vi "ShowInstrParams.vi"(4 "queue out":refnum<queue>, 6 "user event out":refnum<user-event>, 8 "error in (no error)":errorcluster caption="entrée d'erreur (pas d'erreur)", 10 "InstrParam":string, 11 "Experiment en entrée":refnum<class "Experiment.lvclass"> caption="DNL_LabVIEW Object in") -> (0 "error out":errorcluster caption="sortie d'erreur", 3 "Experiment en sortie":refnum<class "Experiment.lvclass"> caption="DNL_LabVIEW Object out")   [LabVIEW 2019, in "Experiment.lvclass"]
uses:
  Experiment.lvclass
  Experiment.lvclass/Experiment.ctl
  DevicesClass/BaseDevice/BaseDevice.lvclass
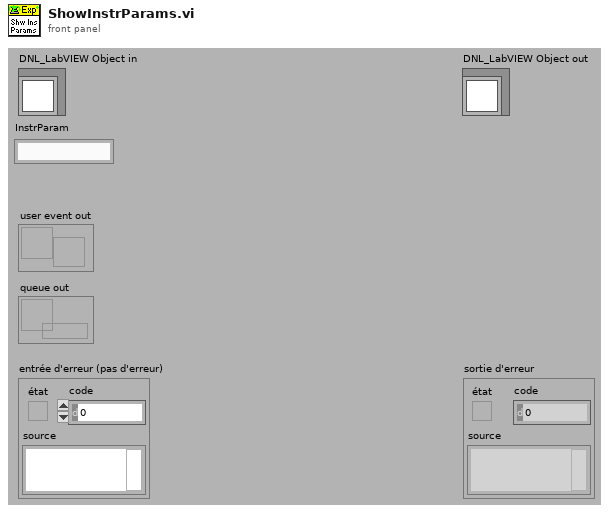
[diagram p1: front panel]
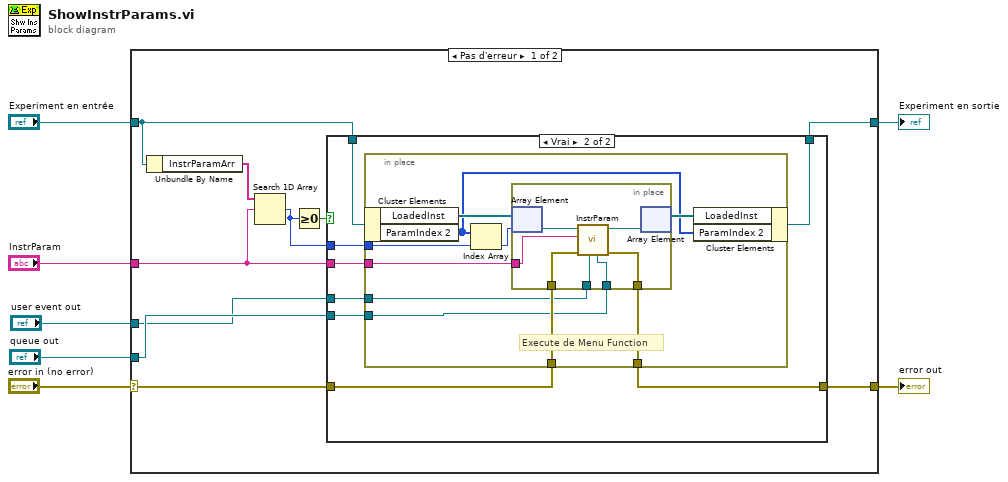
[diagram p0: block diagram]
diagram:
  n1 = case shown="Pas d'erreur" "error in (no error)" {
    selector: "error in (no error)" -> [w15 w46]
    tunnel: [w14 w46] -> w6
    tunnel: [w13 w45] -> w4
    tunnel: "Experiment en entrée" -> [w17 w45]
    tunnel: "InstrParam" -> [w12 _]
    tunnel: "queue out" -> [w9 _]
    tunnel: "user event out" -> [w8 _]
    frame No Error {
      n2 = Unbundle By Name(w17) -> ("InstrParamArr"=w16:string[])
      n3 = Search 1D Array(1D array=w16, element=w12) -> (index of element=w10:i32)  [unwired: 1 in]
      n4 = Greater Or Equal To 0?(x=w10) -> (x >= 0?=w11:bool)
      n5 = case shown="Vrai" w11 {
        tunnel: w17 -> [w18 w27]
        tunnel: w10 -> [_ w26]
        tunnel: w15 -> [w19 w25]
        tunnel: [w19 w24] -> w14
        tunnel: [w18 w23] -> w13
        tunnel: w12 -> [_ w22]
        tunnel: w9 -> [_ w21]
        tunnel: w8 -> [_ w20]
        frame False {
        }
        frame True {
          n6 = in-place {
            in-place-border: w26 -> [w35]
            in-place-border: w25 -> [w33]
            in-place-border: [w32] -> w24
            in-place-border: w22 -> [w31]
            in-place-border: w21 -> [w29]
            in-place-border: w20 -> [w28]
            # "Execute de Menu Function"
            n7 = in-place-cluster #1(w27) -> ("LoadedInst"=w37:refnum<class "BaseDevice.lvclass">[], "ParamIndex 2"=w30:i32[])
            n8 = Index Array(array=w30, index=w35) -> (element=w34:i32)
            n9 = in-place {
              in-place-border: w33 -> [w42]
              in-place-border: [w41] -> w32
              in-place-border: w31 -> [w40]
              in-place-border: w29 -> [w38]
              in-place-border: w28 -> [w39]
              n10 = in-place-array #2(w37, w34) -> (w44:refnum<class "BaseDevice.lvclass">)
              n11 = call-dynamic "InstrParam.vi"("queue out"=w38, "user event out"=w39, "error in (no error)"=w42, "InstrParam"=w40, "BaseDevice en entrée"=w44) -> ("error out"=w41:errorcluster, "BaseDevice en sortie"=w43:refnum<class "BaseDevice.lvclass">)  [unwired: 5 in]
              n12 = in-place-array #2(w43) -> (w36:refnum<class "BaseDevice.lvclass">[])  [unwired: 1 out]
            }
            n13 = in-place-cluster #1("LoadedInst"=w36, "ParamIndex 2"=w30) -> (w23:refnum<class "Experiment.lvclass">)
          }
        }
      }
    }
    frame Error {
    }
  }
  "error out" <- w6
  "Experiment en sortie" <- w4
